vi "Get All VI Strings from Definition.vi"(4 "error in":errorcluster) -> (0 "error out":errorcluster, 3 "VI Strings":T1[](array[typedef]))   [LabVIEW 2025]
doc: "This VI generates an array of clusters that contain the name of each VI in the <i>Test VI Definition.xml</i> file, followed by all strings defined for each VI. This information is used to assert correct functioning of <b>Export Strings.vi</b>"
uses:
  Element Strings--cluster.ctl
  VI Definition--cluster.ctl
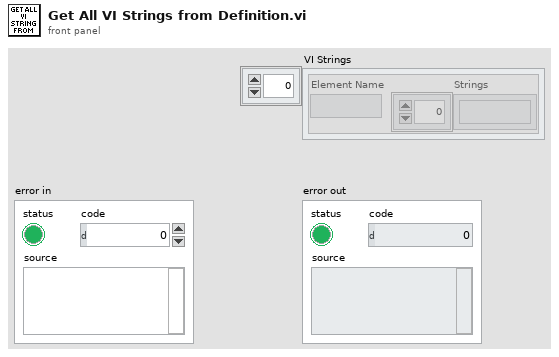
[diagram p1: front panel]
types:
  T1 = typedef "Element Strings--cluster.ctl" = cluster{"Element Name":string, "Strings":string[]}
  T2 = typedef "VI Definition--cluster.ctl" = cluster{"Name":string, "Description":string, "Numeric Indicators":cluster{"Labels":string[]}, "String Controls":cluster{"Labels":string[], "Default Values":string[]}, "Free Labels":cluster{"Text":string[]}, "Front Panel Labels":cluster{"Text":string[]}, "String Constants":cluster{"Text":string[]}}
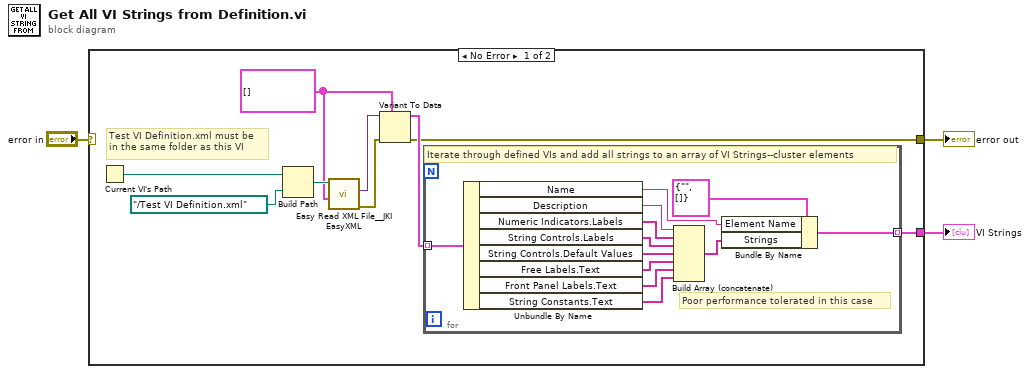
[diagram p0: block diagram]
diagram:
  n1 = case shown="No Error" "error in" {
    selector: "error in" -> [_ w25]
    tunnel: [w4 _] -> w3
    tunnel: [w5 w25] -> w1
    frame No Error {
      w7 = T2[] [] ("Array")
      # "Test VI Definition.xml must be\nin the same folder as this VI"
      n2 = Current VI's Path() -> (path=w12:path)
      n3 = Build Path(base path=w12, name or relative path=path "../Test VI Definition.xml") -> (appended path=w10:path)
      n4 = call <vilib>:"Easy Read XML File__JKI EasyXML.vi"("LabVIEW Data (Type)"=w7, "XML File Path"=w10) -> ("error out"=w8:errorcluster, "LabVIEW Data"=w9:variant)  [unwired: 7 in, 1 out]
      n5 = Variant To Data(error in=w8, type=w7, Variant=w9) -> (data=w6:T2[], error out=w5:errorcluster)
      n6 = for {
        tunnel: w6 -> [w24] mode=indexing
        tunnel: [w13] -> w4 mode=indexing
        # "Poor performance tolerated in this case"
        # "Iterate through defined VIs and add all strings to an array of VI Strings--cluster elements"
        n7 = Unbundle By Name(w24) -> ("Name"=w16:string, "Description"=w23:string, "Numeric Indicators.Labels"=w22:string[], "String Controls.Labels"=w21:string[], "String Controls.Default Values"=w20:string[], "Free Labels.Text"=w19:string[], "Front Panel Labels.Text"=w18:string[], "String Constants.Text"=w17:string[])
        n8 = Build Array (concatenate)(w23, w22, w21, w20, w19, w18, w17) -> (w15:string[])
        n9 = Bundle By Name(cluster=T1 {"Element Name"="", "Strings"=[]} ("VI Strings"), "Element Name"=w16, "Strings"=w15) -> (w13:T1)
      }
    }
    frame Error {
      # "Pass error without  further action"
    }
  }
  "VI Strings" <- w3
  "error out" <- w1
